vi "PicoLog_read.vi"(6 "Conversion":i16 min=0 max=5 step=1, 7 "Single Ended":i16 min=0 max=1 step=1, 9 "Voltage Range":i16 min=0 max=6 step=1, 10 "return type":i16, 11 "Channel":i16=1 min=1 max=16 step=1) -> (1 "Numeric":dbl, 2 "handle":i16, 3 "Over Voltage":i16)   [LabVIEW 2014]
uses:
  PicoHRDL.dll
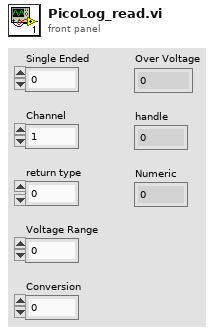
[diagram p1: front panel]
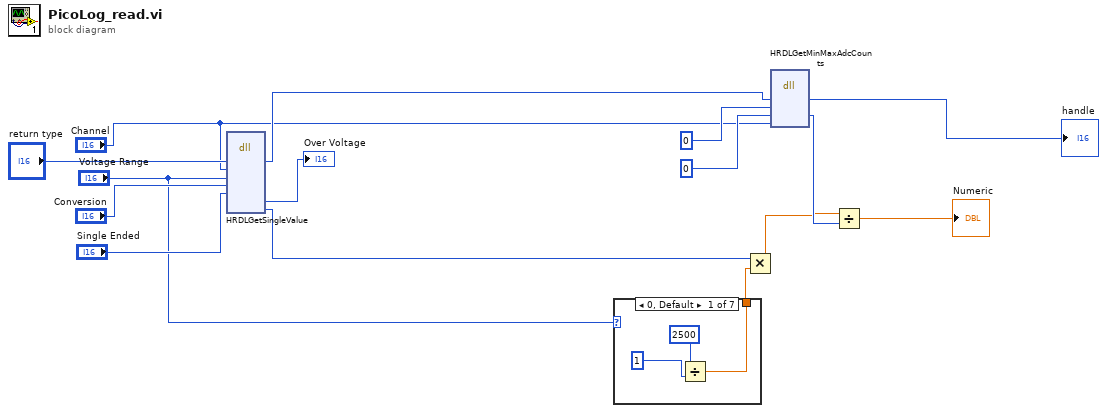
[diagram p0: block diagram]
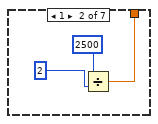
[diagram p2: hidden frame]
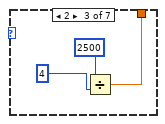
[diagram p3: hidden frame]
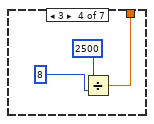
[diagram p4: hidden frame]
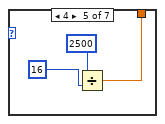
[diagram p5: hidden frame]
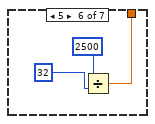
[diagram p6: hidden frame]
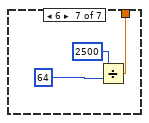
[diagram p7: hidden frame]
diagram:
  n1 = dll-call lib="PicoHRDL.dll" fn="HRDLGetSingleValue"("handle"="return type", "channel"="Channel", "range"="Voltage Range", "conversionTime"="Conversion", "singleEnded"="Single Ended") -> ("handle"=w12:i16, "overflow"=→"Over Voltage":i16, "value"=w14:i32)  [unwired: 10 in, 2 out]
  n2 = case shown="0, Default" "Voltage Range" {
    tunnel: [w16 w19 w22 w25 w28 w31 w34] -> w7
    frame 0, Default {
      n3 = Divide(x=2500, y=1) -> (x/y=w16:dbl)
    }
    frame 1 {
      n4 = Divide(x=2500, y=2) -> (x/y=w19:dbl)
    }
    frame 2 {
      n5 = Divide(x=2500, y=4) -> (x/y=w22:dbl)
    }
    frame 3 {
      n6 = Divide(x=2500, y=8) -> (x/y=w25:dbl)
    }
    frame 4 {
      n7 = Divide(x=2500, y=16) -> (x/y=w28:dbl)
    }
    frame 5 {
      n8 = Divide(x=2500, y=32) -> (x/y=w31:dbl)
    }
    frame 6 {
      n9 = Divide(x=2500, y=64) -> (x/y=w34:dbl)
    }
  }
  n10 = Multiply(x=w14, y=w7) -> (x*y=w8:dbl)
  n11 = dll-call lib="PicoHRDL.dll" fn="HRDLGetMinMaxAdcCounts"("handle"=w12, "minAdc"=0, "maxAdc"=0, "channel"="Channel") -> ("handle"=→"handle":i16, "maxAdc"=w9:i32)  [unwired: 6 in, 2 out]
  n12 = Divide(x=w8, y=w9) -> (x/y=→"Numeric":dbl)
